vi "Format Seqencing Command Pallet.vi"(10 "Paths":path[](array[path]), 11 "Command Info":T4(array[cluster])) -> (2 "Filtered Command Info Out":T1, 3 "2D Picture":picture)   [LabVIEW 2025]
uses:
  <vilib>/picture/picture.llb/imagedata.ctl
  Types/Command Editor Info.ctl
  Types/Single Cmd Info.ctl
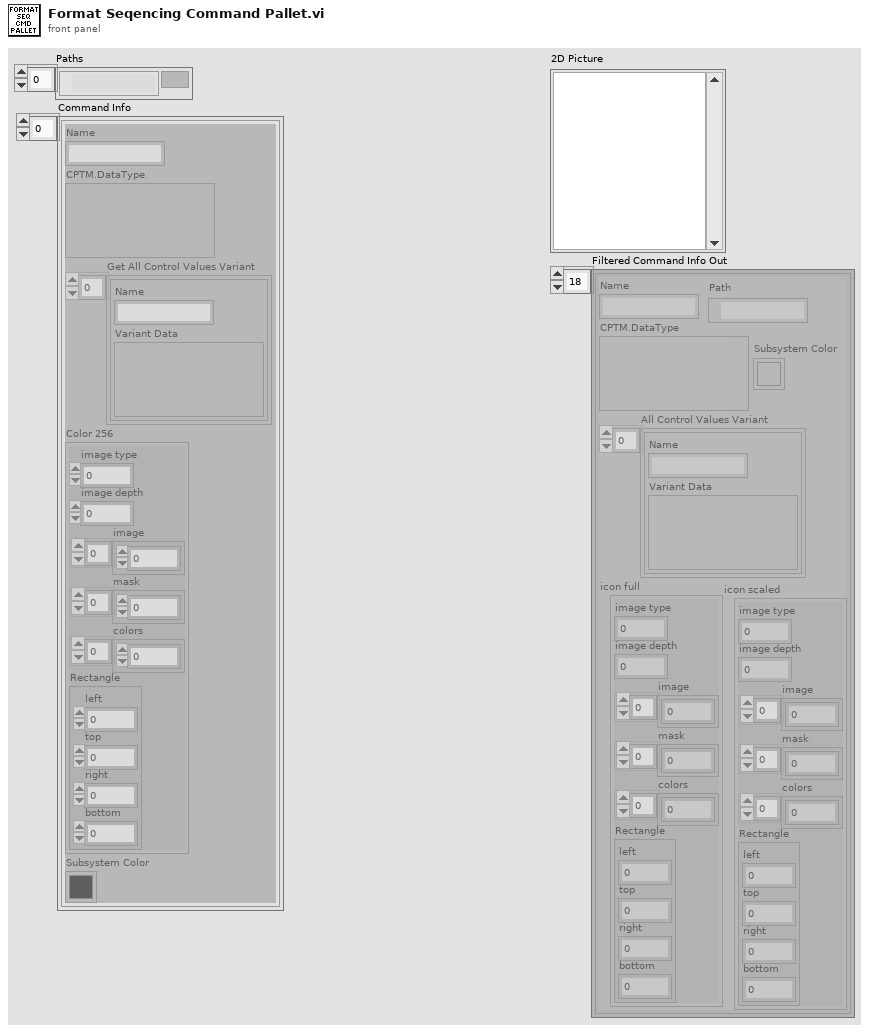
[diagram p1: front panel]
types:
  T1 = typedef "Command Editor Info.ctl" = T2[]
  T2 = typedef "Single Cmd Info.ctl" = cluster{"Name":string, "CPTM.DataType":variant, "All Control Values Variant":cluster{"Name":string, "Variant Data":variant}[], "icon full":T3, "icon scaled":T3, "Path":path, "Subsystem Color":u32}
  T3 = typedef "imagedata.ctl" = cluster{"image type":i32, "image depth":i32, "image":u8[], "mask":u8[], "colors":u32[], "Rectangle":cluster{"left":i16, "top":i16, "right":i16, "bottom":i16}}
  T4 = cluster{"Name":string, "CPTM.DataType":variant, "Get All Control Values Variant":cluster{"Name":string, "Variant Data":variant}[], "Color 256":T3, "Subsystem Color":u32}[]
  T5 = cluster{"Name":string, "CPTM.DataType":variant, "Get All Control Values Variant":cluster{"Name":string, "Variant Data":variant}[], "Color 256":T3, "Color 256":T3, "Path":path, "Subsystem Color":u32}
  T6 = cluster{"left":i16, "top":i16, "right":i16, "bottom":i16}
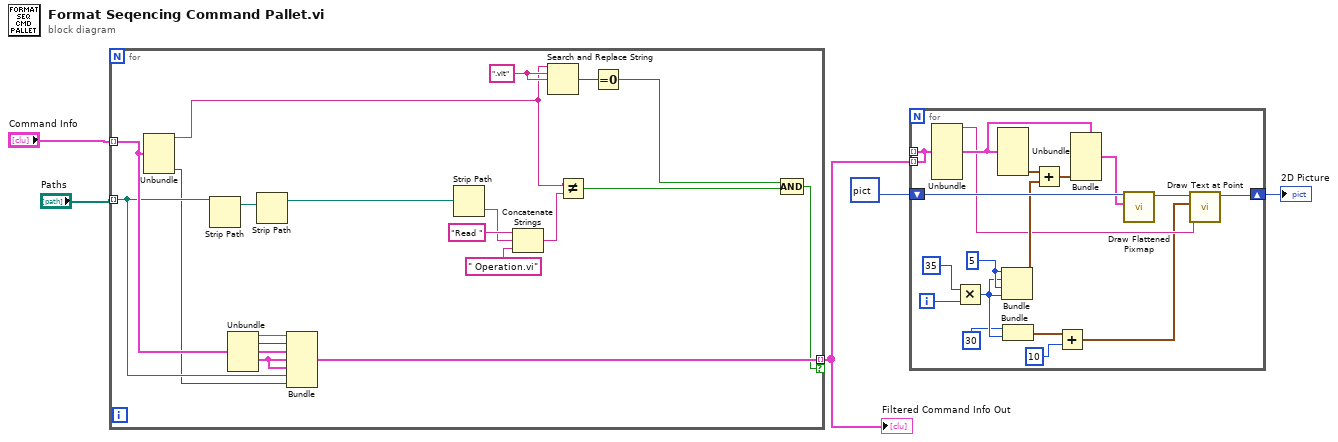
[diagram p0: block diagram]
diagram:
  n1 = for {
    tunnel: "Command Info" -> [w16] mode=indexing
    tunnel: "Paths" -> [w15] mode=indexing
    tunnel: [w17] -> w1 mode=indexing if=w8
    w13 = ".vit" ("search string")
    n2 = Unbundle(w16) -> ("Name"=w6:string, "Subsystem Color"=w14:u32)  [unwired: 3 out]
    n3 = Strip Path(path=w15) -> (stripped path=w25:path)  [unwired: 1 out]
    n4 = Unbundle(w16) -> ("Name"=w18:string, "CPTM.DataType"=w19:variant, "Get All Control Values Variant"=w20:cluster{"Name":string, "Variant Data":variant}[], "Color 256"=w21:T3)  [unwired: 1 out]
    n5 = Strip Path(path=w25) -> (stripped path=w24:path)  [unwired: 1 out]
    n6 = Bundle("Name"=w18, "CPTM.DataType"=w19, "Get All Control Values Variant"=w20, "Color 256"=w21, "Color 256"=w21, "Path"=w15, "Subsystem Color"=w14) -> (w17:T5)  [unwired: 1 in]
    n7 = Strip Path(path=w24) -> (name=w7:string)  [unwired: 1 out]
    n8 = Concatenate Strings("Read ", w7, " Operation.vi") -> (w10:string)
    n9 = Search and Replace String(input string=w6, search string=w13, replace string=w13) -> (number of replacements=w12:i32)  [unwired: 5 in, 3 out]
    n10 = Not Equal?(x=w6, y=w10) -> (x != y?=w9:bool)
    n11 = Equal To 0?(x=w12) -> (x = 0?=w11:bool)
    n12 = Compound Arithmetic op=AND(w11, w9) -> (w8:bool)
  }
  "Filtered Command Info Out" <- w1
  n13 = for {
    tunnel: [w26] -> _ mode=indexing
    shift-right: [w34] -> w2
    shift-left: picture data[5B] ("2D Picture") -> [w43]
    tunnel: w1 -> [w26] mode=indexing
    i -> [w39]
    w38 = 5
    n14 = Unbundle(w26) -> ("Name"=w30:string, "Color 256"=w42:T3)  [unwired: 5 out]
    n15 = Multiply(x=35, y=w39) -> (x*y=w32:i32)
    n16 = Unbundle(w42) -> ("Rectangle"=w40:T6)  [unwired: 5 out]
    n17 = Bundle(w38, w32, w38, w32) -> (w37:cluster{i32, i32, i32, i32})  [unwired: 1 in]
    n18 = Bundle(30, w32) -> (w29:cluster{i32, i32})  [unwired: 1 in]
    n19 = Add(x=w40, y=w37) -> (x+y=w36:cluster{i32, i32, i32, i32})
    n20 = Add(x=w29, y=10) -> (x+y=w28:cluster{i32, i32})
    n21 = Bundle(cluster=w42, "Rectangle"=w36) -> (w41:T3)  [unwired: 5 in]
    n22 = call <vilib>:"Draw Flattened Pixmap.vi"("image data"=w41, "picture"=w43) -> ("new picture"=w35:picture)  [unwired: 7 in]
    n23 = call <vilib>:"Draw Text at Point.vi"("text"=w30, "origin"=w28, "picture"=w35) -> ("new picture"=w34:picture)  [unwired: 7 in, 1 out]
  }
  "2D Picture" <- w2
